vi "DMM initialization.vi"(2 "error in (no error)":errorcluster {"code" format="%.0x"}, 3 "VISA resource name":refnum<visa-resource-name>) -> (0 "error out":errorcluster {"code" format="%.0x"}, 1 "VISA resource name out":refnum<visa-resource-name>)   [LabVIEW 2015]
uses:
  <instrlib>/Hameg DMM/Hameg DMM.lvlib
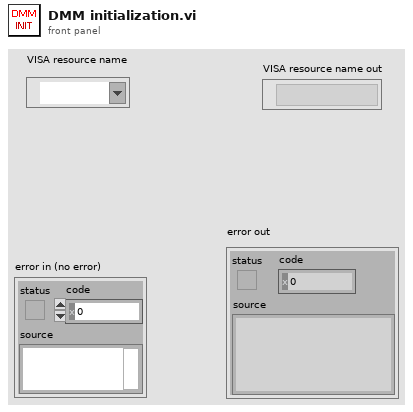
[diagram p1: front panel]
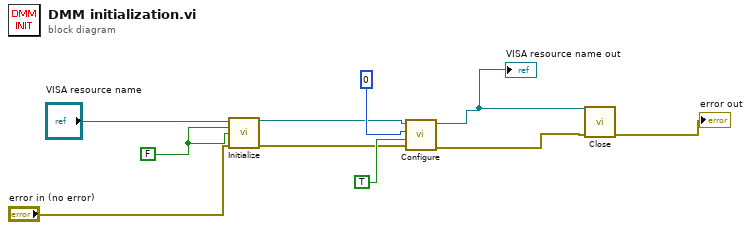
[diagram p0: block diagram]
diagram:
  w6 = FALSE
  n1 = call <instrlib>:"Initialize.vi"("VISA resource name"="VISA resource name", "ID Query (T: Check)"=w6, "Reset (T: Reset)"=w6, "error in (no error)"="error in (no error)") -> ("VISA resource name out"=w5:refnum<visa-resource-name>, "error out"=w4:errorcluster)  [unwired: 10 in]
  n2 = call <instrlib>:"Configure.vi"("error in (no error)"=w4, "Autorange (T: On)"=TRUE, "Function (0: DC Voltage)"=0, "VISA resource name"=w5) -> ("error out"=w2:errorcluster, "VISA resource name out"=w1:refnum<visa-resource-name>)  [unwired: 6 in]
  "VISA resource name out" <- w1
  n3 = call <instrlib>:"Close.vi"("error in (no error)"=w2, "VISA resource name"=w1) -> ("error out"=→"error out":errorcluster)  [unwired: 9 in]
